vi "CBR_Player.vi"() -> ()   [LabVIEW 2014]
panel:
  out "ComType":T1(ring)
  out "Reply":string
  out "file error":errorcluster
  out "connection\nerror":errorcluster
  out "error out":errorcluster
  out "text":string
  in  "Vireo":path=path "/Kim/Users/crogers/Documents/LabVIEW Data/LVVIAGenerated/Demo1.vi  2013-12-18 14-09-36.via"
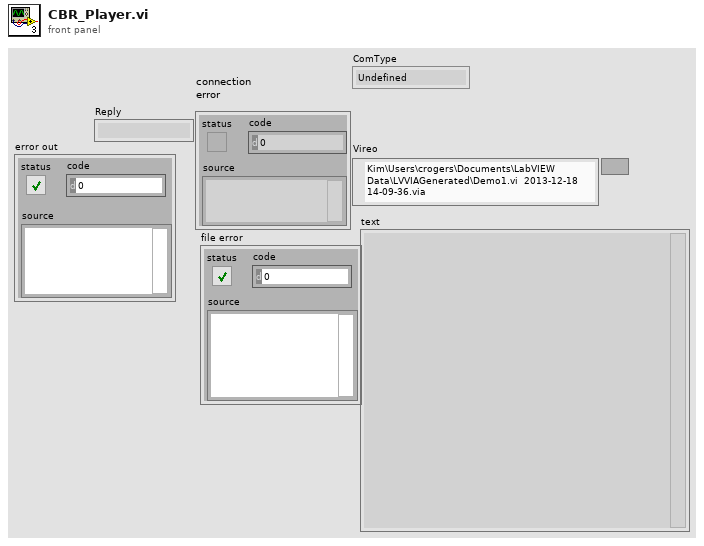
[diagram p1: front panel]
types:
  T1 = enum16{"Undefined", "HTTP", "Serial", "TCPIP", "Console"}
  T2 = typedef "BotSpeak_Control.ctl" = cluster{"Address":string, "Reply EOF":string, "Hardware":string, "Retries":i8, "Timeout":i32, "Open?":bool}
  T3 = typedef "BotSpeak.HardwareSpecs.ctl" = cluster{"Hardware Name":string, "Hardware URL":string, "ComType":enum16{"Undefined", "HTTP", "Serial", "TCPIP", "Console"}, "TCP Port":i32, "DefaultAddress":string, "Retries":i32, "Translate":enum16{"None", "Tiny", "URAPI"}, "MaxScriptSize":i32, "MaxVarNumber":i32, "StartupWait":i32, "Patience":i32, "Startup Patience":i32, "Hardware Help":string, "Com Protocol":string, "Translator":cluster{"BotSpeak CMD":string, "CMD out":string}[], "Init Code":string, "Variable Format":enum16{"INT", "FLOAT", "FIXED"}, "username":string, "password":string}
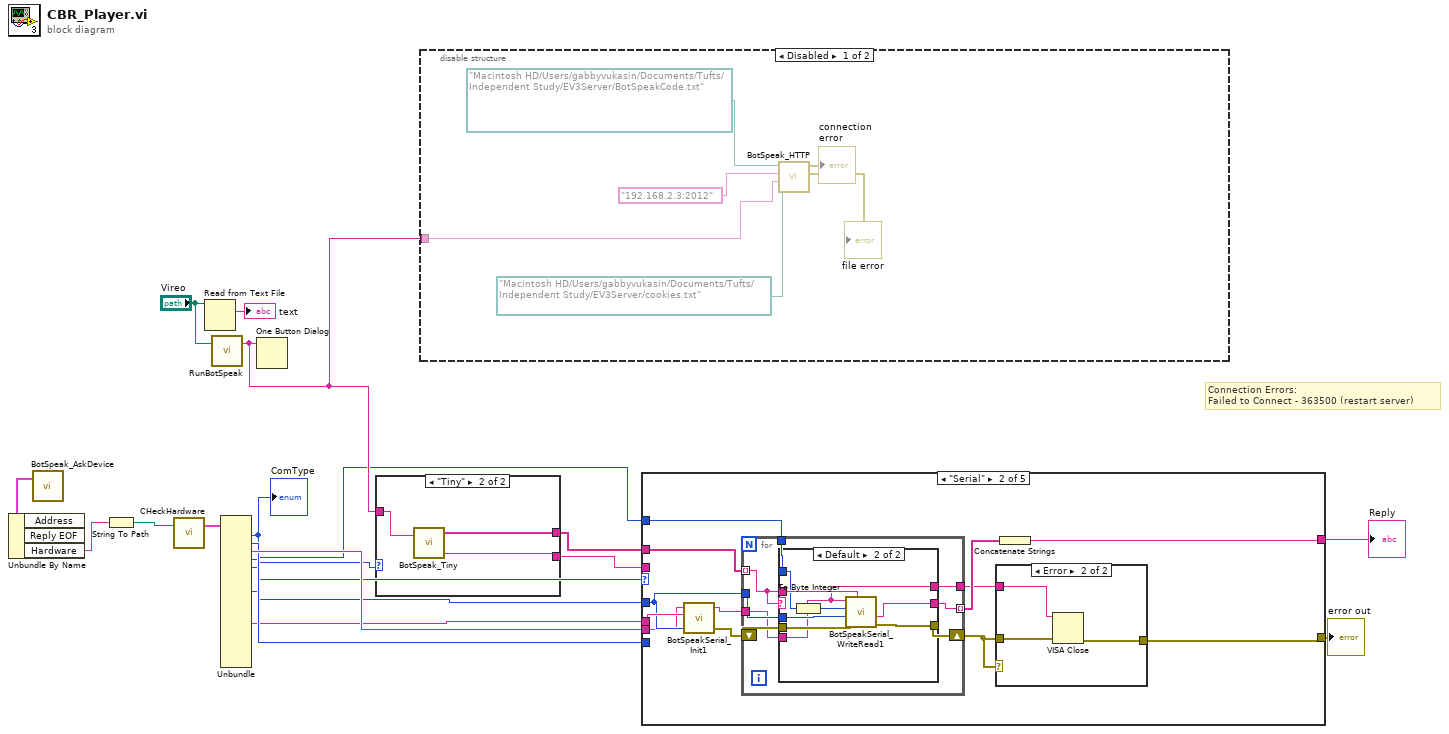
[diagram p0: block diagram]
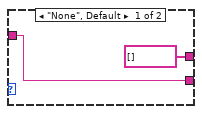
[diagram p2: hidden frame]
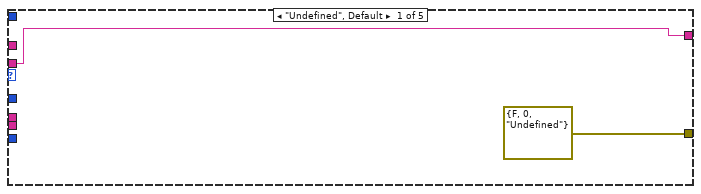
[diagram p3: hidden frame]
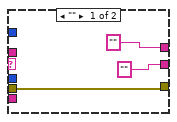
[diagram p4: hidden frame]
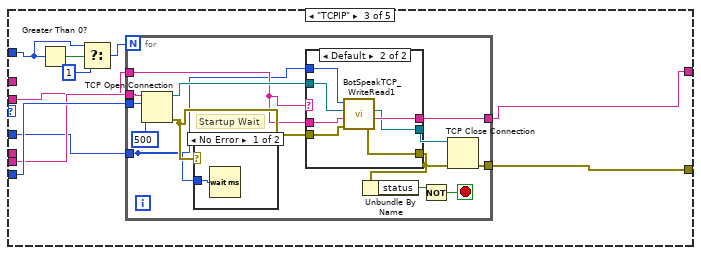
[diagram p6: hidden frame]
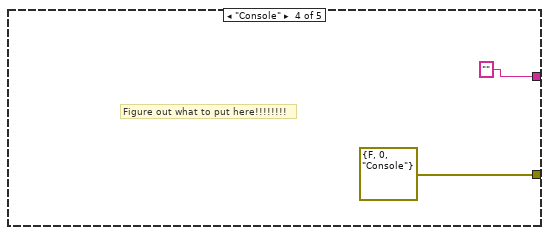
[diagram p9: hidden frame]
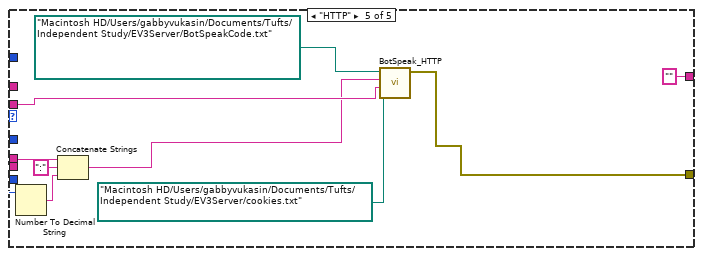
[diagram p10: hidden frame]
diagram:
  # "Connection Errors:\nFailed to Connect - 363500 (restart server)"
  n1 = call <userlib>:"BotSpeak_AskDevice.vi"() -> ("Bot Settings out"=w4:T2)  [unwired: 3 in]
  n2 = Unbundle By Name(w4) -> ("Hardware"=w3:string)  [unwired: 2 out]
  n3 = String To Path(string=w3) -> (path=w5:path)
  n4 = call <userlib>:"CHeckHardware.vi"("Hardware"=w5) -> ("HardwareSpecs"=w9:T3)  [unwired: 2 in]
  n5 = Read from Text File(file (use dialog)="Vireo") -> (text=→"text":string)  [unwired: 3 in, 3 out]
  n6 = call <vilib>:"RunBotSpeak.vi"("VIA"="Vireo") -> ("BotSpeak"=w16:string)  [unwired: 2 in]
  n7 = Unbundle(w9) -> ("ComType"=w8:T1, "TCP Port"=w14:i32, "DefaultAddress"=w15:string, "Retries"=w11:i32, "Translate"=w13:enum16{"None", "Tiny", "URAPI"}, "StartupWait"=w10:i32, "Com Protocol"=w7:string)  [unwired: 12 out]
  "ComType" <- w8
  n8 = One Button Dialog(message=w16) -> ()  [unwired: 1 in, 1 out]
  n9 = case shown="\"Tiny\"" w13 {
    tunnel: w16 -> [w20 w23]
    tunnel: [w20 w22] -> w12
    tunnel: [string[] [] ("Tiny Lines") w21] -> w1
    frame "None", Default {
    }
    frame "Tiny" {
      n10 = call <userlib>:"BotSpeak_Tiny.vi"("URAPI"=w23) -> ("URAPI  2"=w22:string, "Tiny Lines"=w21:string[])  [unwired: 1 in, 1 out]
    }
  }
  n11 = disable-structure shown="Disabled" {
    disable-tunnel: w16 -> [w26 _]
    frame Disabled {
      n12 = call <userlib>:"BotSpeak_HTTP.vi"("BotSpeak File Name"=path "/Macintosh HD/Users/gabbyvukasin/Documents/Tufts/Independent Study/EV3Server/BotSpeakCode.txt", "URL"="192.168.2.3:2012", "BotSpeak Code"=w26, "cookie file"=path "/Macintosh HD/Users/gabbyvukasin/Documents/Tufts/Independent Study/EV3Server/cookies.txt") -> ("connection\nerror"=→"connection\nerror":errorcluster, "file error"=→"file error":errorcluster)  [unwired: 5 in]
    }
    frame Enabled {
    }
  }
  n13 = case shown="\"Serial\"" w8 {
    tunnel: w12 -> [w30 _ w68 _ w109]
    tunnel: w15 -> [_ w35 w70 _ w108]
    tunnel: w14 -> [_ _ w71 _ w106]
    tunnel: w11 -> [_ w40 w73 _ _]
    tunnel: w10 -> [_ w39 w69 _ _]
    tunnel: w7 -> [_ w42 _ _ _]
    tunnel: [errorcluster {"status"=FALSE, "code"=0, "source"="Undefined"} ("connection\nerror") w38 w67 errorcluster {"status"=FALSE, "code"=0, "source"="Console"} ("connection\nerror") w103] -> w6
    tunnel: [w30 w33 w66 "" ("Reply") "" ("Reply")] -> w2
    tunnel: w1 -> [_ w36 _ _ _]
    frame "Undefined", Default {
    }
    frame "Serial" {
      n14 = call <userlib>:"BotSpeakSerial_Init1.vi"("StartupWait"=w39, "Com Protocol"=w42, "Address"=w35) -> ("error out"=w41:errorcluster)  [unwired: 2 in]
      n15 = for {
        tunnel: w40 -> [w49]
        tunnel: w39 -> [w48]
        shift-right: [w47] -> w37
        shift-left: w41 -> [w50]
        tunnel: w36 -> [w46] mode=indexing
        tunnel: [w45] -> w34 mode=indexing
        tunnel: w35 -> [w44]
        tunnel: [w43] -> w32
        n16 = case shown="Default" w46 {
          tunnel: w50 -> [w53 w61]
          tunnel: [w53 w60] -> w47
          tunnel: w46 -> [_ w59]
          tunnel: w44 -> [_ w54]
          tunnel: w49 -> [_ w56]
          tunnel: w48 -> [_ w58]
          tunnel: ["" ("Reply") w55] -> w45
          tunnel: ["" ("DefaultAddress") w54] -> w43
          frame "" {
          }
          frame Default {
            n17 = To Byte Integer(number=w56) -> (8bit integer=w57:i8)
            n18 = call <userlib>:"BotSpeakSerial_WriteRead1.vi"("To Write"=w59, "error In"=w61, "Timeout"=w58, "Retries"=w57, "Address"=w54) -> ("error out"=w60:errorcluster, "Reply"=w55:string)  [unwired: 1 in, 1 out]
          }
        }
      }
      n19 = case shown="Error" w37 {
        tunnel: [w62 w65] -> w38
        tunnel: w37 -> [w62 w64]
        tunnel: w32 -> [_ w63]
        frame No Error {
          # "Should this \nclose anyway?"
        }
        frame Error {
          n20 = VISA Close(VISA resource name=w63, error in (no error)=w64) -> (error out=w65:errorcluster)
        }
      }
      n21 = Concatenate Strings(w34) -> (w33:string)
    }
    frame "TCPIP" {
      n22 = Greater Than 0?(x=w73) -> (x > 0?=w75:bool)
      n23 = Select(t=w73, s=w75, f=1) -> (s? t:f=w74:i32)
      n24 = for {
        N: w74 -> [_]
        tunnel: w71 -> [w88]
        tunnel: w70 -> [w86]
        tunnel: w69 -> [w80]
        tunnel: w68 -> [w83]
        tunnel: [w82] -> w66
        tunnel: [w79] -> w67
        stop <- w76 stop-if-true
        # "Startup Wait"
        n25 = TCP Open Connection(address=w86, remote port or service name=w88, timeout ms (60000)=500) -> (connection ID=w85:refnum<k5>, error out=w84:errorcluster)  [unwired: 2 in]
        n26 = case shown="No Error" w84 {
          tunnel: w80 -> [w99 _]
          frame No Error {
            n27 = Wait (ms)(milliseconds to wait=w99) -> ()  [unwired: 1 out]
          }
          frame Error {
          }
        }
        n28 = case shown="Default" w83 {
          tunnel: w85 -> [w90 w98]
          tunnel: w83 -> [w91 w97]
          tunnel: [w91 w96] -> w82
          tunnel: w84 -> [w89 w95]
          tunnel: [w90 w94] -> w81
          tunnel: [w89 w93] -> w78
          tunnel: w80 -> [_ w92]
          frame "" {
          }
          frame Default {
            n29 = call <userlib>:"BotSpeakTCP_WriteRead1.vi"("error in"=w95, "To Send"=w97, "connection ID"=w98, "Timeout"=w92) -> ("error out"=w93:errorcluster, "data out"=w96:string, "connection ID out"=w94:refnum<k5>)  [unwired: 1 in]
          }
        }
        n30 = Unbundle By Name(w78) -> ("status"=w77:bool)
        n31 = Not(x=w77) -> (.not. x?=w76:bool)
        n32 = TCP Close Connection(connection ID=w81, error in (no error)=w78) -> (error out=w79:errorcluster)  [unwired: 1 in, 1 out]
      }
    }
    frame "Console" {
      # "Figure out what to put here!!!!!!!!"
    }
    frame "HTTP" {
      n33 = Number To Decimal String(number=w106) -> (decimal integer string=w105:string)  [unwired: 1 in]
      n34 = Concatenate Strings(w108, ":" ("string"), w105) -> (w104:string)
      n35 = call <userlib>:"BotSpeak_HTTP.vi"("BotSpeak File Name"=path "/Macintosh HD/Users/gabbyvukasin/Documents/Tufts/Independent Study/EV3Server/BotSpeakCode.txt", "URL"=w104, "BotSpeak Code"=w109, "cookie file"=path "/Macintosh HD/Users/gabbyvukasin/Documents/Tufts/Independent Study/EV3Server/cookies.txt") -> ("connection\nerror"=w103:errorcluster)  [unwired: 5 in, 1 out]
    }
  }
  "error out" <- w6
  "Reply" <- w2
